vi "Is equal.vi"(4 "other address":refnum<class "Generic Network Address.lvclass">, 5 "address":refnum<class "Generic Network Address.lvclass">) -> (1 "equal?":bool)   [LabVIEW 2020, in "NI_WFCN.lvlib" / "Generic Network Address.lvclass"]
doc: "Returns TRUE if the addresses are equal."
uses:
  <vilib>/net/WFCN/Addressing/Generic Network Address/Generic Network Address.lvclass
  <vilib>/net/WFCN/Addressing/Generic Network Address/Generic Network Address.lvclass/Generic Network Address.ctl
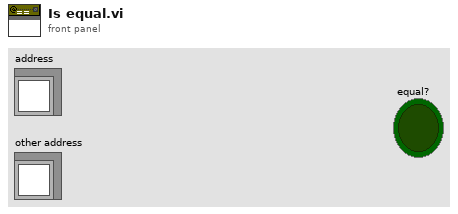
[diagram p1: front panel]
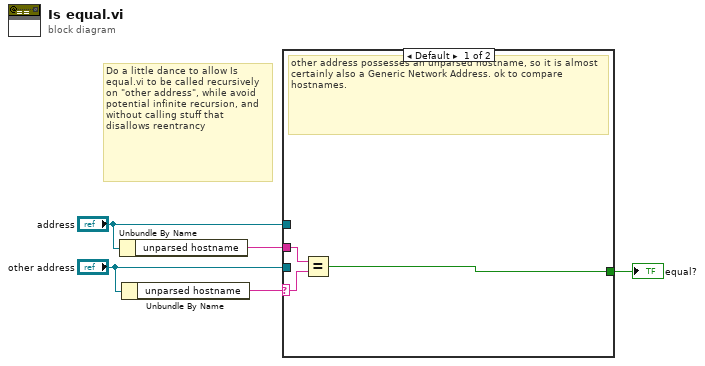
[diagram p0: block diagram]
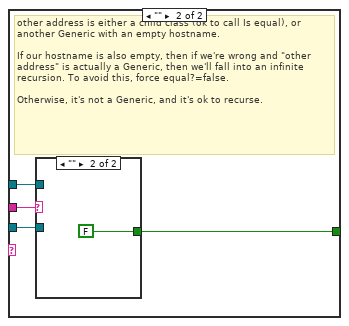
[diagram p2: hidden frame]
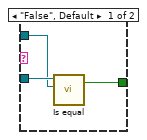
[diagram p3: hidden frame]
diagram:
  # "Do a little dance to allow Is equal.vi to be called recursively on \"other address\", while avoid potential infinite recursion, and without calling stuff that disallows reentrancy"
  n1 = Unbundle By Name("address") -> ("unparsed hostname"=w5:string)
  n2 = Unbundle By Name("other address") -> ("unparsed hostname"=w4:string)
  n3 = case shown="Default" w4 {
    selector: w4 -> [w7 _]
    tunnel: w5 -> [w8 w12]
    tunnel: "address" -> [_ w9]
    tunnel: [w6 w11] -> w2
    tunnel: "other address" -> [_ w10]
    frame Default {
      # "other address possesses an unparsed hostname, so it is almost certainly also a Generic Network Address. ok to compare hostnames."
      n4 = Equal?(x=w8, y=w7) -> (x = y?=w6:bool)
    }
    frame "" {
      # "other address is either a child class (ok to call Is equal), or another Generic with an empty hostname.\n\nIf our hostname is also empty, then if we're wrong and \"other address\" is actually a Generic, then we'll fall into an infinite recursion. To avoid this, force equal?=false.\n\nOtherwise, it's not a Generic, and it's ok to recurse."
      n5 = case shown="\"\"" w12 {
        tunnel: [w13 FALSE] -> w11
        tunnel: w10 -> [w15 _]
        tunnel: w9 -> [w14 _]
        frame "False", Default {
          n6 = call-dynamic "Is equal.vi"("other address"=w14, "address"=w15) -> ("equal?"=w13:bool)  [unwired: 3 in]
        }
        frame "" {
        }
      }
    }
  }
  "equal?" <- w2
